vi "crc16-ccitt (x1021).vi"(8 "error in (no error)":errorcluster, 10 "unsigned byte array":u8[](array[numeric])=[96, 8, 128, 86]) -> (0 "error out (dup)":errorcluster, 2 "CRC":u8[](array[numeric]))   [LabVIEW 2009]
doc: "This VI takes in a string variable and calculates the 16-bit CRC value based on the CRC16-CCITT standard (polynomial 0x1021) with seed value of 0xFFFF ONLY!!!\n\nThis VI code is based on an extremely efficient implementation originally intended for microcontrollers and is adapted for LabVIEW. All thanks go to:\nOriginal Code: Ashley Roll\nOptimisations: Scott Dattalo"
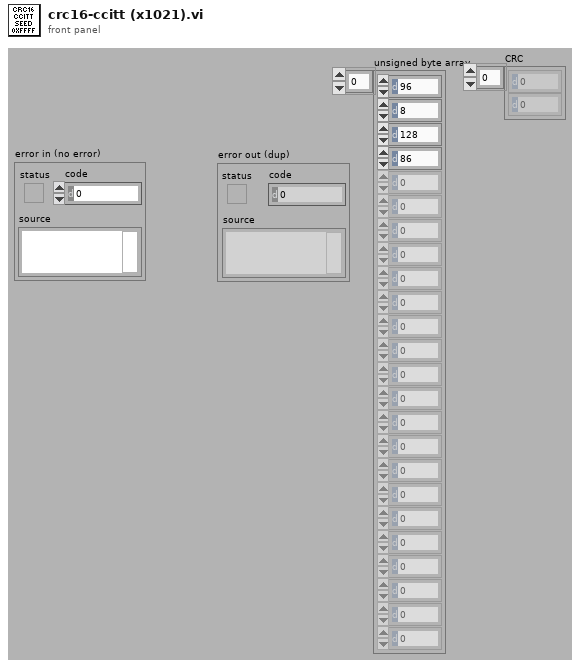
[diagram p1: front panel]
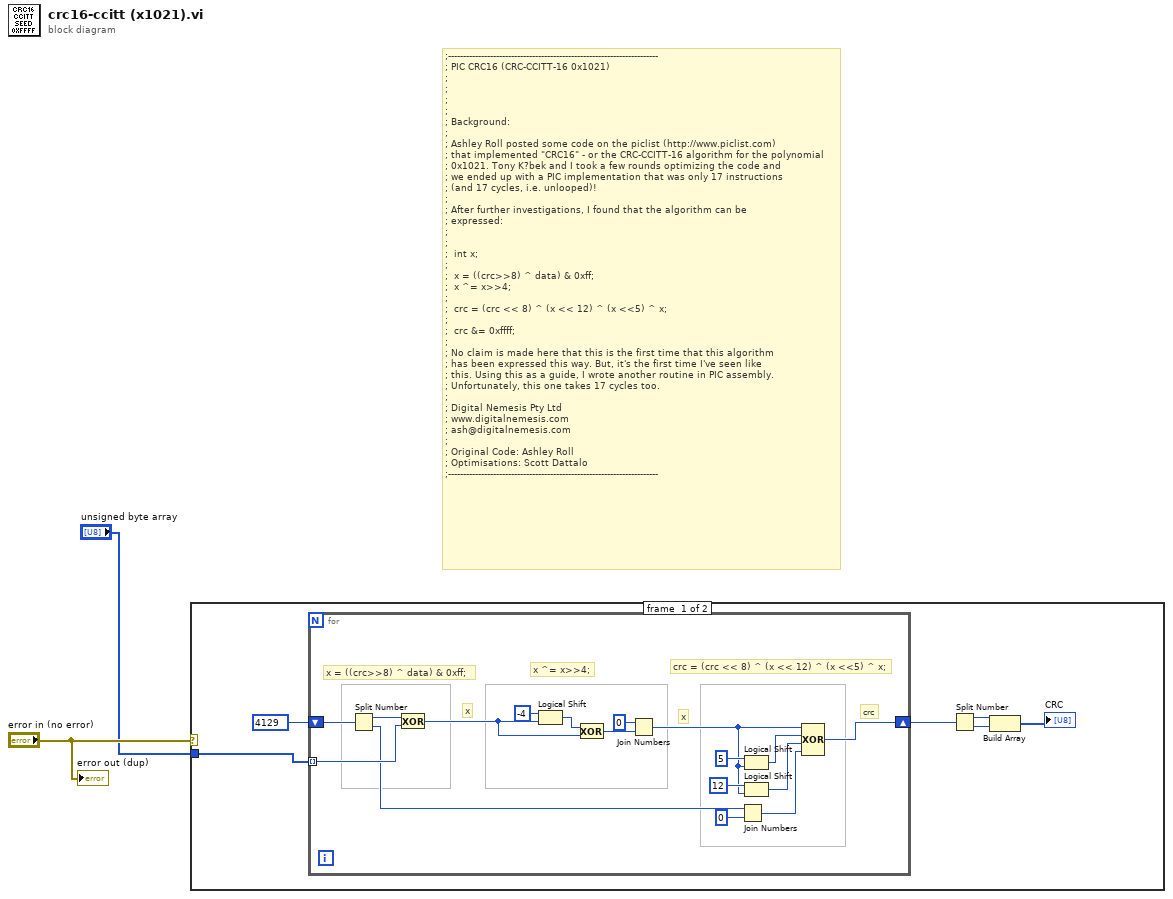
[diagram p0: block diagram]
diagram:
  # ";----------------------------------------------------------------------\n; PIC CRC16 (CRC-CCITT-16 0x1021)\n;\n;\n; \n;\n; Background:\n;\n; Ashley Roll posted some code on the piclist (http://www.piclist.com)\n; that implemented \"CRC16\" - or the CRC-CCITT-16 algorithm for the polynomial\n; 0x1021. Tony K?bek and I took a few rounds optimizing the code and\n; we ended up with a PIC implementation that was only 17 instructions\n; (and 17 cycles, i.e. unlooped)!\n;\n; After further investigations, I found that the algorithm can be \n; expressed:\n;\n;\n;  int x;\n;\n;  x = ((crc>>8) ^ data) & 0xff;\n;  x ^= x>>4;\n;\n;  crc = (crc << 8) ^ (x << 12) ^ (x <<5) ^ x;\n;\n;  crc &= 0xffff;\n;\n; No claim is made here that this is the first time that this algorithm\n; has been expressed this way. But, it's the first time I've seen like\n; this. Using this as a guide, I wrote another routine in PIC assembly.\n; Unfortunately, this one takes 17 cycles too.\n;\n; Digital Nemesis Pty Ltd\n; www.digitalnemesis.com\n; ash@digitalnemesis.com\n;\n; Original Code: Ashley Roll\n; Optimisations: Scott Dattalo\n;----------------------------------------------------------------------"
  n1 = case shown="No Error" "error in (no error)" {
    tunnel: "unsigned byte array" -> [w7 _]
    frame #0 {
      n2 = for {
        tunnel: w7 -> [w19] mode=indexing
        shift-right: [w9] -> w6
        shift-left: u16 4129 -> [w18]
        # "crc"
        # "crc = (crc << 8) ^ (x << 12) ^ (x <<5) ^ x;"
        # "x"
        # "x ^= x>>4;"
        # "x"
        # "x = ((crc>>8) ^ data) & 0xff;"
        n3 = Split Number(x=w18) -> (hi(x)=w25:u8, lo(x)=w12:u8)
        n4 = Exclusive Or(1:w19, 2:w25) -> (0:w22:u8)
        n5 = Logical Shift(y=i8 -4, x=w22) -> (x << y=w23:u8)
        n6 = Exclusive Or(1:w22, 2:w23) -> (0:w21:u8)
        n7 = Join Numbers(hi=u8 0, lo=w21) -> ((hi.lo)=w14:u16)
        n8 = Join Numbers(hi=w12, lo=u8 0) -> ((hi.lo)=w10:u16)
        n9 = Logical Shift(y=i8 5, x=w14) -> (x << y=w16:u16)
        n10 = Logical Shift(y=i8 12, x=w14) -> (x << y=w13:u16)
        n11 = Compound Arithmetic op=XOR(w14, w16, w13, w10) -> (w9:u16)
      }
      n12 = Split Number(x=w6) -> (hi(x)=w5:u8, lo(x)=w4:u8)
      n13 = Build Array(w5, w4) -> (→"CRC":u8[])
    }
    frame #1 {
    }
  }
  "error out (dup)" <- "error in (no error)"
